vi "Activate Logic.vi"(10 "Deactivate":bool, 11 "Activate":bool) -> (3 "Output":bool)   [LabVIEW 2015, in "SLZ-KA1 Actor.lvlib" / "SLZ-KA1.lvclass"]
doc: "Set output to <b>TRUE</b> if Output was <b>TRUE</b> or Activate is a rising edge and Deactivate is <b>FALSE</b>."
uses:
  SLZ-KA1.lvclass
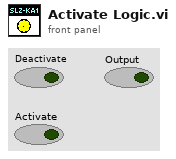
[diagram p1: front panel]
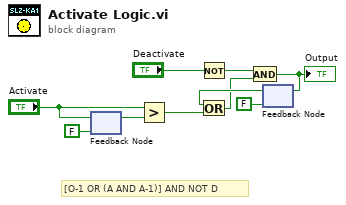
[diagram p0: block diagram]
diagram:
  # "[O-1 OR (A AND A-1)] AND NOT D"
  n1 = feedback #1(FALSE ("Boolean")) -> (w9:bool)
  n2 = feedback-in #1("Activate") -> ()
  n3 = Greater?(x="Activate", y=w9) -> (0:w10:bool)
  n4 = Not(x="Deactivate") -> (.not. x?=w6:bool)
  n5 = feedback #2(FALSE) -> (w4:bool)
  n6 = Or(x=w4, y=w10) -> (x .or. y?=w2:bool)
  n7 = And(x=w6, y=w2) -> (x .and. y?=w5:bool)
  "Output" <- w5
  n8 = feedback-in #2(w5) -> ()
